vi "DCMotor.vi"() -> ()   [LabVIEW 2018]
uses:
  <vilib>/MakerHub/LINX/Public/Utilities/Open Serial.vi
  <vilib>/MakerHub/LINX/Public/Sensors/Motion/Servo/Servo Open One Channel.vi
  <vilib>/MakerHub/LINX/Public/Sensors/Motion/Servo/Servo Set Pulse Width One Channel.vi
  <vilib>/MakerHub/LINX/Public/Sensors/Motion/Servo/Servo Close One Channel.vi
  <vilib>/MakerHub/LINX/LMH-LINX.lvlib
  <vilib>/MakerHub/LINX/Public/Sensors/Motion/Servo/Servo.lvlib
panel:
  in  "Speed RPM":dbl(knob) scale=-100.0..100.0
  in  "Servo Channel":u8
  in  "?":bool
  in  "Baud Rate Override":u32
  in  "Serial Port":refnum<visa-resource-name>="N/A"
  # "Arduino Settings"
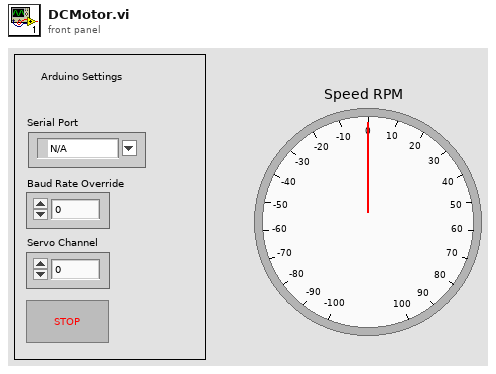
[diagram p1: front panel]
types:
  T1 = typedef "LMH-LINX.lvlib/LINX Ref.ctl" = cluster{"IO":T2, "Interface":T3, "LINX Device Config":T4}
  T2 = typedef "LMH-LINX.lvlib/Platform.ctl" = enum16{"Remote", "Local"}
  T3 = typedef "LMH-LINX.lvlib/Interface.ctl" = enum16{"Serial", "TCP"}
  T4 = typedef "LMH-LINX.lvlib/Device.lvlib/LINX Device Config.ctl" = cluster{"Interface":T3, "COM Port":refnum<visa-resource-name>, "TCP Configuration":T5, "Device Family":u8, "Device ID":u8, "Device Name":string, "TCP Ref":refnum<k5>, "Channels":T6}
  T5 = typedef "LMH-LINX.lvlib/Device.lvlib/TCP Config.ctl" = cluster{"IP Address":string, "Port":u16}
  T6 = typedef "LMH-LINX.lvlib/Channels.ctl" = cluster{"DI":u8[], "DO":u8[], "AI":u8[], "AO":u8[], "PWM":u8[], "QE":u8[], "UART":u8[], "I2C 2":u8[], "SPI":u8[], "CAN":u8[], "Servo":u8[], "AI Ref (V)":dbl, "AI Resolution (Bits)":u8, "AO Ref (V)":dbl, "AO Resolution (Bits)":u8}
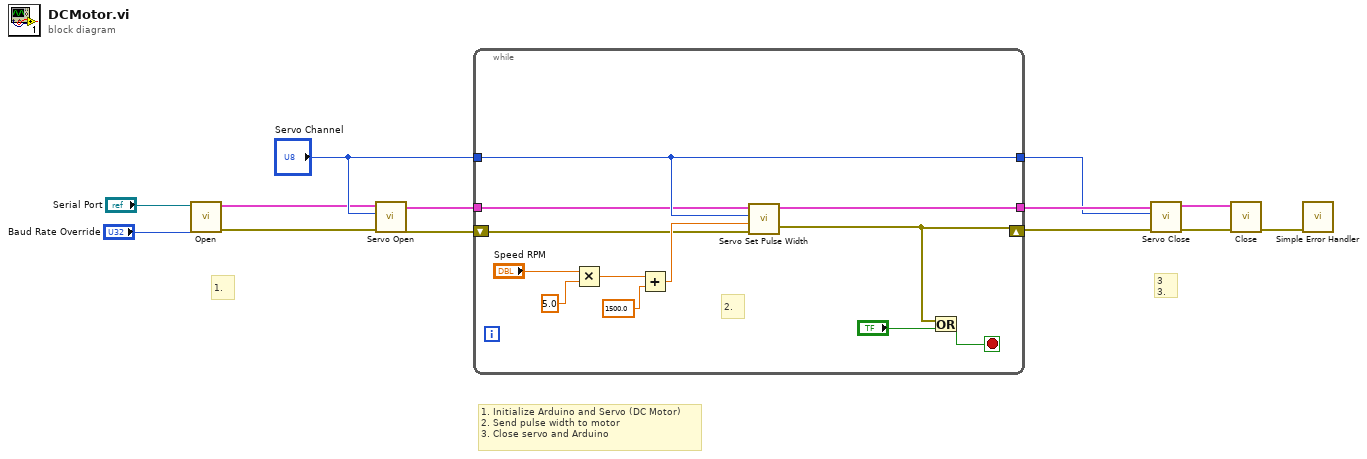
[diagram p0: block diagram]
diagram:
  # "1. Initialize Arduino and Servo (DC Motor)\n2. Send pulse width to motor\n3. Close servo and Arduino"
  # "3\n3."
  # "1."
  n1 = call-poly <vilib>:"Open.vi"("Baud Rate Override"="Baud Rate Override", "Serial Port"="Serial Port") -> ("Error Out"=w1:errorcluster, "LINX Resource"=w2:T1)  [unwired: 7 in, 1 out]
  n2 = call-poly <vilib>:"Servo Open.vi"("Error In"=w1, "Servo Channel"="Servo Channel", "LINX Resource"=w2) -> ("Error Out"=w9:errorcluster, "LINX Resource"=w10:T1)  [unwired: 7 in]
  n3 = while {
    tunnel: w10 -> [w16]
    tunnel: [w25] -> w8
    shift-right: [w14] -> w7
    shift-left: w9 -> [w15]
    tunnel: "Servo Channel" -> [w24]
    tunnel: [w24] -> w3
    stop <- w22 stop-if-true
    # "2."
    n4 = Multiply(x="Speed RPM", y=5.0) -> (x*y=w21:dbl)
    n5 = Add(x=w21, y=1500.0) -> (x+y=w17:dbl)
    n6 = call-poly <vilib>:"Servo Set Pulse Width.vi"("Error In"=w15, "Pulse Width (uS)"=w17, "Servo Channel"=w24, "LINX Resource"=w16) -> ("Error Out"=w14:errorcluster, "LINX Resource"=w25:T1)  [unwired: 6 in]
    n7 = Or(x=w14, y="?") -> (x .or. y?=w22:bool)
  }
  n8 = call-poly <vilib>:"Servo Close.vi"("Error In"=w7, "Servo Channel"=w3, "LINX Resource"=w8) -> ("Error Out"=w5:errorcluster, "LINX Resource"=w6:T1)  [unwired: 7 in]
  n9 = call <vilib>:"Close.vi"("Error In"=w5, "LINX Resource"=w6) -> ("Error Out"=w11:errorcluster)  [unwired: 9 in]
  n10 = call <vilib>:"Simple Error Handler.vi"("error in (no error)"=w11) -> ()  [unwired: 4 in, 5 out]
